vi "Nanosleep Absolute (seconds).vi"(8 "error in (no error)":errorcluster, 10 "clock id (monotonic)":T1=enum."Monotonic", 11 "sleep until (seconds)":dbl=1000000000.0) -> (0 "error out":errorcluster, 3 "current time (seconds)":dbl=1000000000.0)   [LabVIEW 2013, in "Linux RT Utilities.lvlib"]
uses:
  Linux RT Utilities.lvlib
  Controls/Public/C Enums/clockid_t.ctl
  Controls/Public/nanosleep flags.ctl
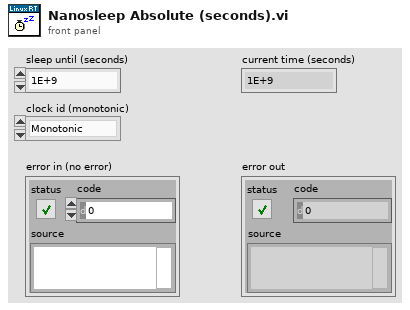
[diagram p1: front panel]
types:
  T1 = typedef "Linux RT Utilities.lvlib/clockid_t.ctl" = enum16{"Realtime", "Monotonic"}
  T2 = typedef "Linux RT Utilities.lvlib/nanosleep flags.ctl" = enum16{"Relative Time", "Absolute Time"}
  T3 = typedef "Linux RT Utilities.lvlib/timespec_64.ctl" = cluster{"sec":u64, "nsec":u64}
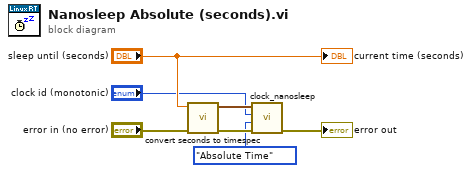
[diagram p0: block diagram]
diagram:
  n1 = call "convert seconds to timespec.vi"("seconds"="sleep until (seconds)") -> ("timespec"=w3:T3)  [unwired: 10 in]
  n2 = call "clock_nanosleep.vi"("error in (no error)"="error in (no error)", "flags"=nanosleep_flags."Absolute Time", "clockid_t"="clock id (monotonic)", "request"=w3) -> ("error out"=→"error out":errorcluster)  [unwired: 6 in, 1 out]
  "current time (seconds)" <- "sleep until (seconds)"
